vi "18BitTo20Bit.vi"(4 "18Bit":i32 format="%018b") -> (1 "20Bit":i32 format="%020b")   [LabVIEW 2014]
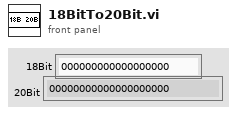
[diagram p1: front panel]
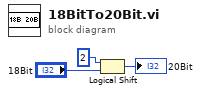
[diagram p0: block diagram]
diagram:
  n1 = Logical Shift(y=i16 2, x="18Bit") -> (x << y=→"20Bit":i32)
